vi "test log.vi"() -> ()   [LabVIEW 2017]
panel:
  in  "file path (use dialog)":path
  in  "Stop Button":bool
  out "String":string
  in  "Action to run":T1(ring)
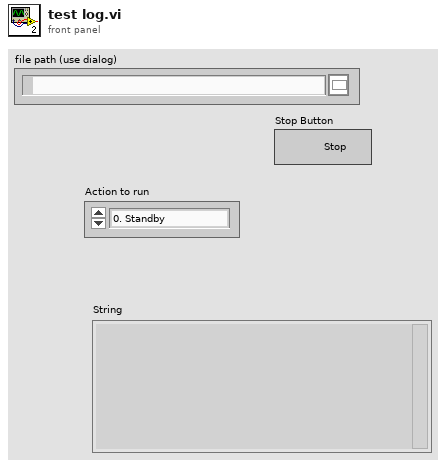
[diagram p1: front panel]
types:
  T1 = enum16{"0. Standby", "1. Purge with Argon", "2. Rinse with solvent", "3. Prepare droplet", "4. Reaction"}
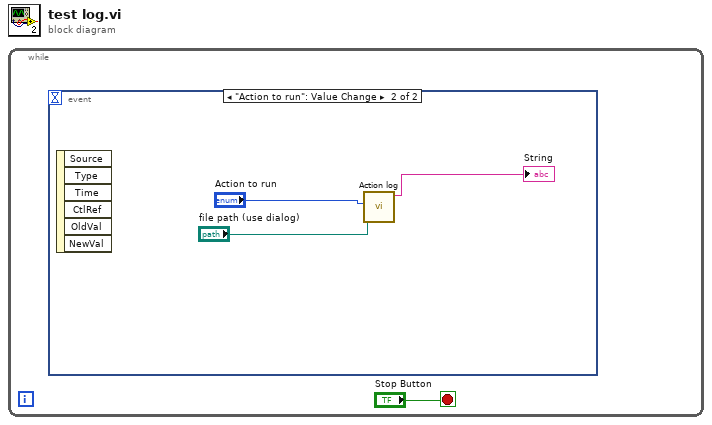
[diagram p0: block diagram]
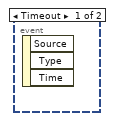
[diagram p2: hidden frame]
diagram:
  n1 = while {
    stop <- "Stop Button" stop-if-true
    n2 = event shown="[1] \"Action to run\": Value Change" {
      selector: _ -> [_ _]
      dyn-events: _ -> [_ _]
      timeout: _ -> [_ _]
      event Timeout {
        n3 = event-data() -> ()  [unwired: 1 in, 3 out]
      }
      event "Action to run": Value Change {
        n4 = event-data() -> ()  [unwired: 1 in, 6 out]
        n5 = call "Action log.vi"("file path (use dialog)"="file path (use dialog)", "Action running"="Action to run") -> ("Action log out"=→"String":string)  [unwired: 8 in, 1 out]
      }
    }
  }
